vi "Get Event DVR.vi"(11 "Hello World Event in":refnum<class "Hello World Event.lvclass">) -> (2 "Event Self":map{string, refnum<data-value>}(c390))   [LabVIEW 2021, in "Hello World Event.lvlib" / "Hello World Event.lvclass"]
uses:
  Hello World Event.lvclass
  Hello World Event.lvclass/Hello World Event.ctl
  Actor/Event Actor/Event Actor.lvclass
  Actor/Msg/Msg.lvclass
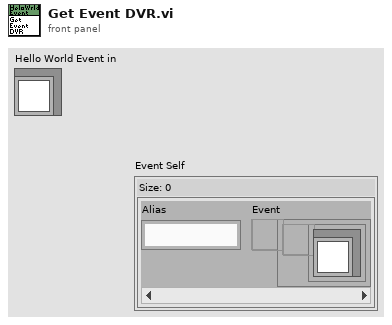
[diagram p1: front panel]
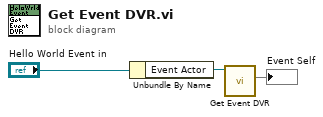
[diagram p0: block diagram]
diagram:
  n1 = Unbundle By Name("Hello World Event in") -> ("Event Actor"=w2:refnum<class "Event Actor.lvclass">)
  n2 = call-dynamic "Get Event DVR.vi"("Event Actor in"=w2) -> ("Event Self"=→"Event Self":map{string, refnum<data-value>})  [unwired: 10 in]
